vi "Cannon Sensors Update.vi"(1 "Cannon Info In":T2) -> (0 "Cannon Info Out":T2)   [LabVIEW 2013]
uses:
  <vilib>/Rock Robotics/WPI/Relay/WPI_RelayValue.ctl
  Cannon Global.vi
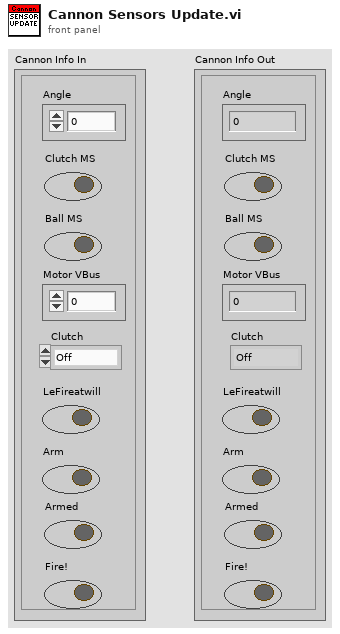
[diagram p1: front panel]
types:
  T1 = typedef "WPI_RelayValue.ctl" = enum16{"Off", "On", "Forward", "Reverse"}
  T2 = cluster{"Angle":dbl, "Clutch MS":bool, "Ball MS":bool, "Motor VBus":dbl, "Clutch ":T1, "LeFireatwill":bool, "Arm":bool, "Armed":bool, "Fire!":bool}
  T3 = typedef "WPI_AnalogChannelDevRef.ctl" = cluster{"DevStatus":errorcluster, "Analog Module":T4, "Analog Channel":T5}
  T4 = typedef "FPGA_TypedefAnalogModule.ctl" = enum16{"Analog Module 1", "Analog Module 2"}
  T5 = typedef "FPGA_AIChannel.ctl" = enum8{"AI 1", "AI 2", "AI 3", "AI 4", "AI 5", "AI 6", "AI 7", "AI 8", "Invalid"}
  T6 = typedef "WPI_DigitalInputDevRef.ctl" = cluster{"DevStatus":errorcluster, "DIO Channel":T7, "Digital Module":T8}
  T7 = typedef "FPGA_DIOChannel.ctl" = enum8{"DIO 1", "DIO 2", "DIO 3", "DIO 4", "DIO 5", "DIO 6", "DIO 7", "DIO 8", "DIO 9", "DIO 10", "DIO 11", "DIO 12", "DIO 13", "DIO 14", "Invalid"}
  T8 = typedef "FPGA_TypedefDigitalModule.ctl" = enum16{"Digital Module 1", "Digital Module 2"}
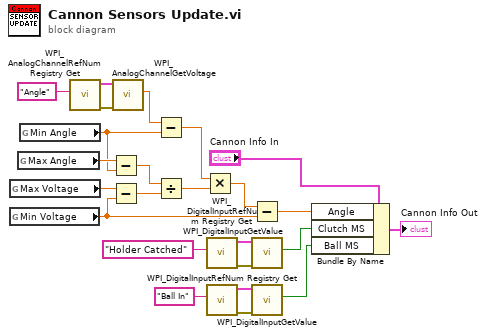
[diagram p0: block diagram]
diagram:
  n1 = global read "Cannon Global.vi" "Max Voltage"() -> (w18:dbl)
  n2 = global read "Cannon Global.vi" "Min Voltage"() -> (w10:dbl)
  n3 = global read "Cannon Global.vi" "Max Angle"() -> (w19:dbl)
  n4 = global read "Cannon Global.vi" "Min Angle"() -> (w14:dbl)
  n5 = call <vilib>:"WPI_AnalogChannelRefNum Registry Get.vi"("refnum name"="Angle") -> ("error out"=w21:errorcluster, "AIDeviceRef"=w20:T3)  [unwired: 9 in]
  n6 = Subtract(x=w19, y=w14) -> (x-y=w17:dbl)
  n7 = Subtract(x=w18, y=w10) -> (x-y=w16:dbl)
  n8 = call <vilib>:"WPI_AnalogChannelGetVoltage.vi"("error in (no error)"=w21, "AIDeviceRef"=w20) -> ("Voltage"=w13:dbl)  [unwired: 7 in, 2 out]
  n9 = Subtract(x=w13, y=w14) -> (x-y=w12:dbl)
  n10 = Divide(x=w17, y=w16) -> (x/y=w15:dbl)
  n11 = Multiply(x=w12, y=w15) -> (x*y=w11:dbl)
  n12 = call <vilib>:"WPI_DigitalInputRefNum Registry Get.vi"("refnum name"="Holder Catched") -> ("error out"=w8:errorcluster, "DigitalInputDevRef"=w7:T6)  [unwired: 9 in]
  n13 = call <vilib>:"WPI_DigitalInputRefNum Registry Get.vi"("refnum name"="Ball In") -> ("error out"=w5:errorcluster, "DigitalInputDevRef"=w4:T6)  [unwired: 9 in]
  n14 = Subtract(x=w11, y=w10) -> (x-y=w9:dbl)
  n15 = call <vilib>:"WPI_DigitalInputGetValue.vi"("error in (no error)"=w8, "DigitalInputDevRef"=w7) -> ("Value"=w6:bool)  [unwired: 7 in, 2 out]
  n16 = call <vilib>:"WPI_DigitalInputGetValue.vi"("error in (no error)"=w5, "DigitalInputDevRef"=w4) -> ("Value"=w3:bool)  [unwired: 7 in, 2 out]
  n17 = Bundle By Name(cluster="Cannon Info In", "Angle"=w9, "Clutch MS"=w6, "Ball MS"=w3) -> (→"Cannon Info Out":T2)
